vi "avToShortSpectrumAv.vi"(1 "attribute value":T1={"device name"="", "attribute name"="", "quality value"=enum."VALID", "quality string"="", "timestamp"=0.0, "dim. x"=0, "dim. y"=0, "value"=[], "error code"=0, "error stack"=[], "data type"=enum."UNKNOWN_DATA_TYPE"}) -> (0 "av":T4={"device name"="", "attribute name"="", "quality value"=0, "quality string"="", "timestamp"=0.0, "dim. x"=0, "dim. y"=0, "value"=[], "error code"=0, "error stack"=[], "data type"=36})   [LabVIEW 2014, in "tango.lvlib"]
uses:
  tango.lvlib
  Common VIs/Typedefs/_AttributeValue_t.ctl
  Common VIs/Typedefs/_AttributeQuality_t.ctl
  Common VIs/Typedefs/_AttributeDataType_t.ctl
  base/toShortSpectrum.vi
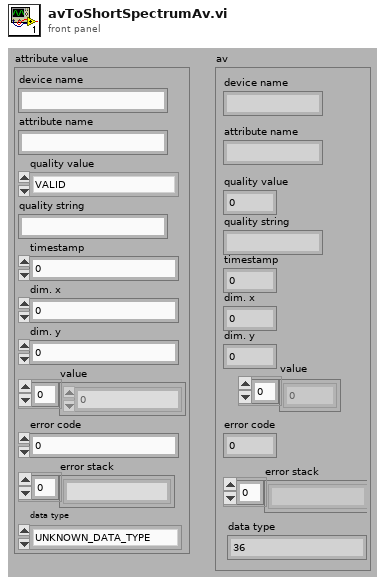
[diagram p1: front panel]
types:
  T1 = typedef "tango.lvlib/_AttributeValue_t.ctl" = cluster{"device name":string, "attribute name":string, "quality value":T2, "quality string":string, "timestamp":dbl, "dim. x":i32, "dim. y":i32, "value":u8[], "error code":i32, "error stack":string[], "data type":T3}
  T2 = typedef "tango.lvlib/_AttributeQuality_t.ctl" = enum16{"VALID", "INVALID", "ALARM", "CHANGING", "UNKNOWN_QUALITY"}
  T3 = typedef "tango.lvlib/_AttributeDataType_t.ctl" = enum16{"STATE_SCA", "STATE_SPE", "STATE_IMG", "STRING_SCA", "STRING_SPE", "STRING_IMG", "BOOL_SCA", "BOOL_SPE", "BOOL_IMG", "UCHAR_SCA", "UCHAR_SPE", "UCHAR_IMG", "SHORT_SCA", "SHORT_SPE", "SHORT_IMG", "USHORT_SCA", "USHORT_SPE", "USHORT_IMG", "LONG_SCA", "LONG_SPE", "LONG_IMG", "ULONG_SCA", "ULONG_SPE", "ULONG_IMG", "LONG64_SCA", "LONG64_SPE", "LONG64_IMG", "ULONG64_SCA", "ULONG64_SPE", "ULONG64_IMG", "FLOAT_SCA", "FLOAT_SPE", "FLOAT_IMG", "DOUBLE_SCA", "DOUBLE_SPE", "DOUBLE_IMG", "UNKNOWN_DATA_TYPE"}
  T4 = cluster{"device name":string, "attribute name":string, "quality value":i16, "quality string":string, "timestamp":dbl, "dim. x":i32, "dim. y":i32, "value":i16[], "error code":i32, "error stack":string[], "data type":u16}
  T5 = cluster{"device name":string, "attribute name":string, "quality value":T2, "quality string":string, "timestamp":dbl, "dim. x":i32, "dim. y":i32, "value_out":i16[], "error code":i32, "error stack":string[], "data type":T3}
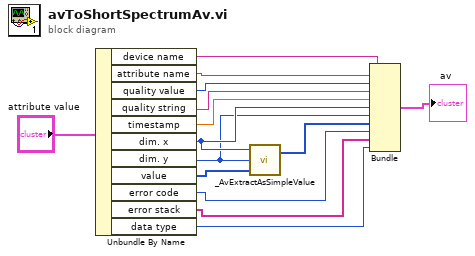
[diagram p0: block diagram]
diagram:
  n1 = Unbundle By Name("attribute value") -> ("device name"=w13:string, "attribute name"=w12:string, "quality value"=w11:T2, "quality string"=w10:string, "timestamp"=w9:dbl, "dim. x"=w8:i32, "dim. y"=w7:i32, "value"=w14:u8[], "error code"=w5:i32, "error stack"=w4:string[], "data type"=w1:T3)
  n2 = call-poly "_AvExtractAsSimpleValue.vi"("value_in"=w14, "dim_y"=w7, "dim_x"=w8) -> ("value_out"=w6:i16[])  [unwired: 1 out]
  n3 = Bundle("device name"=w13, "attribute name"=w12, "quality value"=w11, "quality string"=w10, "timestamp"=w9, "dim. x"=w8, "dim. y"=w7, "value_out"=w6, "error code"=w5, "error stack"=w4, "data type"=w1) -> (→"av":T5)  [unwired: 1 in]
